vi "getAnalogIn.vi"(6 "AnalogIn":sgl, 8 "error in (no error)":errorcluster, 9 "AnalogInId":u8, 10 "Device":i32, 11 "SEDSpectrometer in":refnum<class "SEDSpectrometer.lvclass">) -> (0 "error out":errorcluster, 1 "AnalogIn":sgl, 2 "Output Value":i32, 3 "SEDSpectrometer out":refnum<class "SEDSpectrometer.lvclass">)   [LabVIEW 2016, in "SEDSpectrometer.lvclass"]
uses:
  SEDSpectrometer.lvclass
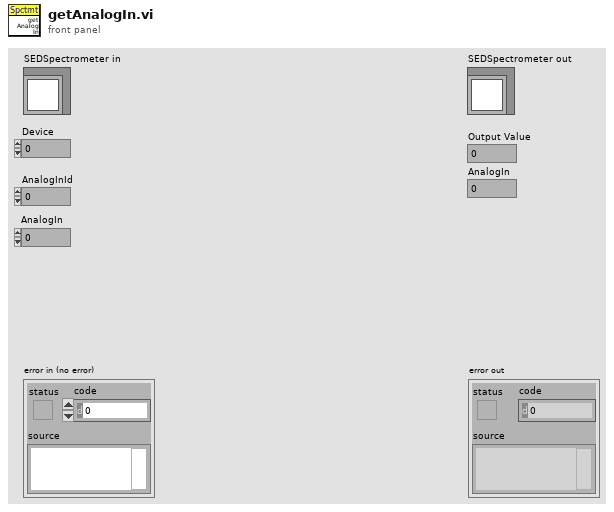
[diagram p1: front panel]
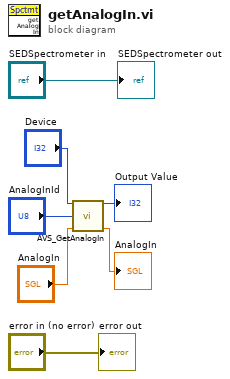
[diagram p0: block diagram]
diagram:
  n1 = call "AVS_GetAnalogIn.vi"("a_hDevice"="Device", "a_AnalogInId"="AnalogInId", "a_pAnalogIn"="AnalogIn") -> ("Output Value"=→"Output Value":i32, "a_pAnalogIn"=→"AnalogIn":sgl)  [unwired: 11 in]
  "error out" <- "error in (no error)"
  "SEDSpectrometer out" <- "SEDSpectrometer in"
